vi "Auto Angle.vi"(9 "Yaw":T10 scale format="%.3f", 10 "Rotation PID Config":T2 {"Max I Accu"."Low" format="%#.8f"; "Max I Accu"."High" format="%#.8f"; "Gains"."F" format="%#.8f"; "Gains"."D" format="%#.8f"; "Gains"."I" format="%#.8f"; "Gains"."P" format="%#.8f"; "Error Allowed"."Low" format="%#.8f"; "Error Allowed"."High" format="%#.8f"; "I Zone"."Low" format="%#.8f"; "I Zone"."High" format="%#.8f"; "Max Out"."REV" format="%.2f"; "Max Out"."FWD" format="%.2f"}, 11 "CMD_ACT_SwerveDrive_Data in":T6 {"Auto Angle" scale format="%.3f"; "Direction"."Rotate(Yaw) CCW 1 CW -1" scale=1.0..-1.0; "Direction"."Traverse"."Angle" scale format="%.3f"; "Direction"."Traverse"."Velocity" scale=-1.0..1.0 scale format="%.1f"}) -> (1 "At Angle":bool, 3 "CMD_ACT_SwerveDrive_Data out":T6 {"Auto Angle" scale format="%.3f"; "Direction"."Rotate(Yaw) CCW 1 CW -1" scale=1.0..-1.0; "Direction"."Traverse"."Angle" scale format="%.3f"; "Direction"."Traverse"."Velocity" scale=-1.0..1.0 scale format="%.1f"})   [LabVIEW 2023, in "Thor-SwerveDrive_ACT.lvlib"]
uses:
  Thor-SwerveDrive_ACT.lvlib
  Shared Code/TypeDefs/Dial_Compase heading unit circle CCW positive.ctl
  Shared Code/TypeDefs/ENUM_Swerve_CMD_Mode Select.ctl
  Shared Code/TypeDefs/Level_Velocity plus-minus 1.ctl
  Shared Code/TypeDefs/Cluster_Module Velocity-Direction-Rotations.ctl
  Type Defs/NUM_Rotate Input.ctl
  Shared Code/TypeDefs/Cluster_CMD_Direction Data.ctl
  Shared Code/TypeDefs/Cluster_X-Y.ctl
  Cluster_CMD_ACT_Data.ctl
  Shared Code/TypeDefs/Cluster_FWD  REV Values.ctl
  Shared Code/TypeDefs/Cluster_High-Low.ctl
  Shared Code/TypeDefs/Cluster_PID Gains.ctl
  Shared Code/TypeDefs/Cluster_PID Config.ctl
panel:
  out "Mode":T1
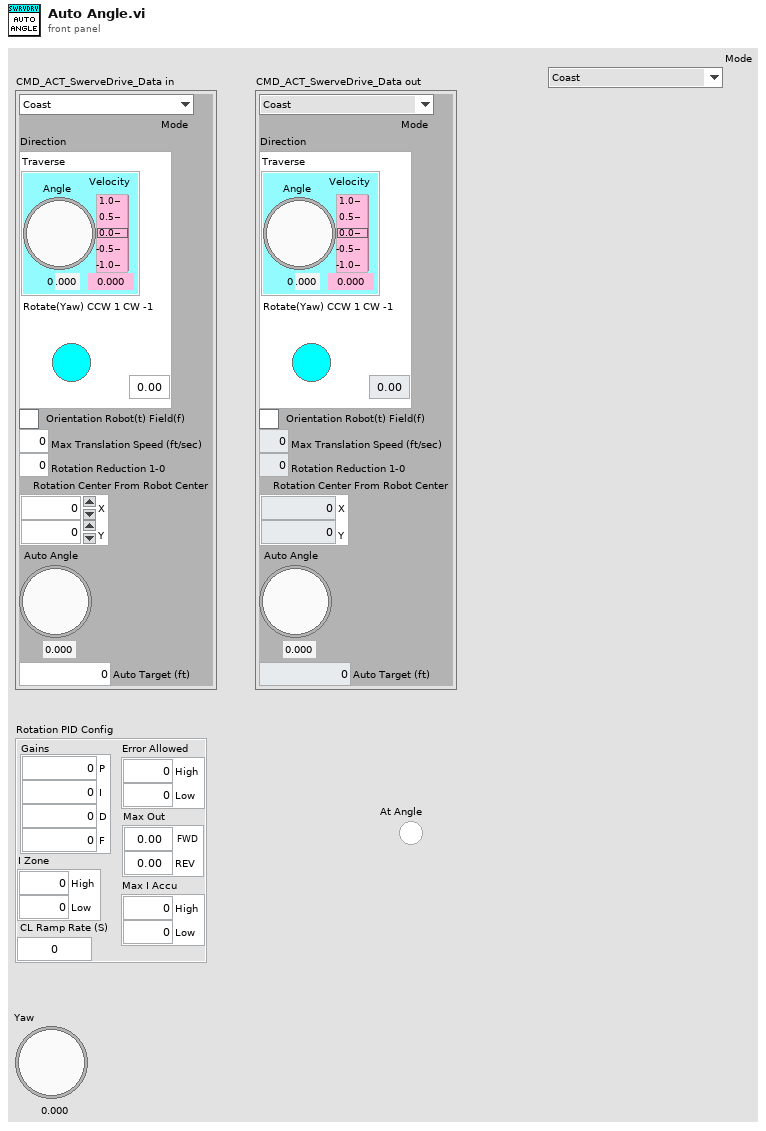
[diagram p1: front panel]
types:
  T1 = typedef "ENUM_Swerve_CMD_Mode Select.ctl" = enum16{"Coast", "Manual", "Auto Trans Auto Rotate", "Manual Trans Auto Rotate", "Balance", "Stop Brake", "Lock Wheels"}
  T2 = typedef "Cluster_PID Config.ctl" = cluster{"Gains":T3, "Error Allowed":T4, "I Zone":T4, "Max Out":T5, "Max I Accu":T4, "CL Ramp Rate (S)":dbl}
  T3 = typedef "Cluster_PID Gains.ctl" = cluster{"P":dbl, "I":dbl, "D":dbl, "F":dbl}
  T4 = typedef "Cluster_High-Low.ctl" = cluster{"High":dbl, "Low":dbl}
  T5 = typedef "Cluster_FWD  REV Values.ctl" = cluster{"FWD":dbl, "REV":dbl}
  T6 = typedef "Thor-SwerveDrive_ACT.lvlib/Cluster_CMD_ACT_Data.ctl" = cluster{"Mode":T1, "Direction":T7, "Orientation Robot(t) Field(f)":bool, "Max Translation Speed (ft/sec)":dbl, "Rotation Reduction 1-0":dbl, "Rotation Center From Robot Center":T12, "Auto Angle":T10, "Auto Target (ft)":dbl}
  T7 = typedef "Cluster_CMD_Direction Data.ctl" = cluster{"Traverse":T8, "Rotate(Yaw) CCW 1 CW -1":T11}
  T8 = typedef "Cluster_Module Velocity-Direction-Rotations.ctl" = cluster{"Velocity":T9, "Angle":T10, "Rotations Count":dbl}
  T9 = typedef "Level_Velocity plus-minus 1.ctl" = dbl
  T10 = typedef "Dial_Compase heading unit circle CCW positive.ctl" = dbl
  T11 = typedef "NUM_Rotate Input.ctl" = dbl
  T12 = typedef "Cluster_X-Y.ctl" = cluster{"X":dbl, "Y":dbl}
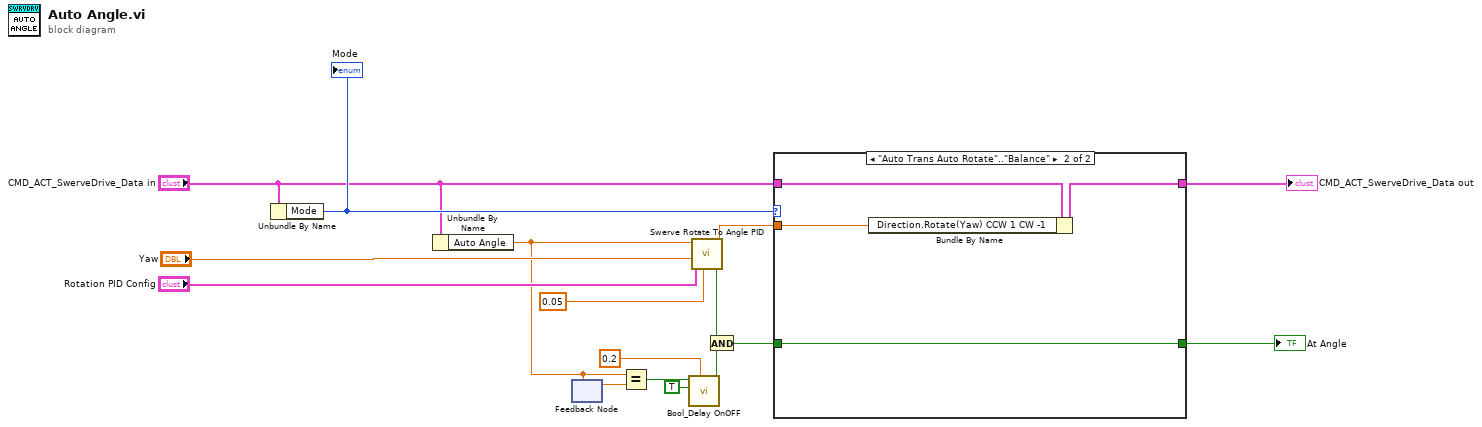
[diagram p0: block diagram]
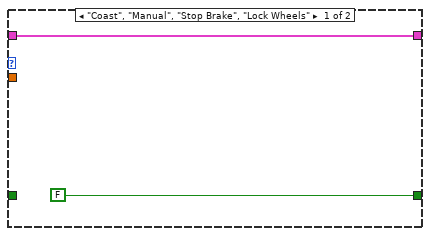
[diagram p2: hidden frame]
diagram:
  n1 = Unbundle By Name("CMD_ACT_SwerveDrive_Data in") -> ("Mode"=w14:T1)
  "Mode" <- w14
  n2 = Unbundle By Name("CMD_ACT_SwerveDrive_Data in") -> ("Auto Angle"=w8:T10)
  n3 = feedback #1() -> (w9:T10)  [unwired: 1 in]
  n4 = feedback-in #1(w8) -> ()
  n5 = Equal?(x=w8, y=w9) -> (x = y?=w7:bool)
  n6 = call "Bool_Delay OnOFF.vi"("Delay Time(S)"=0.2, "Delay On(t) Off(f)"=TRUE, "Input"=w7) -> ("Output"=w4:bool)  [unwired: 7 in, 1 out]
  n7 = call "Swerve Rotate To Angle PID.vi"("Target Cycle Time(S)"=0.05, "PID Config"="Rotation PID Config", "Current Yaw"="Yaw", "Target Yaw"=w8) -> ("At Angle Out"=w3:bool, "Direction.Rotate(Yaw) CCW 1 CW -1 Out"=w10:T11)  [unwired: 5 in, 1 out]
  n8 = And(x=w3, y=w4) -> (x .and. y?=w2:bool)
  n9 = case shown="\"Auto Trans Auto Rotate\"..\"Balance\"" w14 {
    tunnel: "CMD_ACT_SwerveDrive_Data in" -> [w18 w22]
    tunnel: w10 -> [_ w21]
    tunnel: [w18 w20] -> w12
    tunnel: w2 -> [_ w19]
    tunnel: [FALSE w19] -> w1
    frame "Coast", "Manual", "Stop Brake", "Lock Wheels" {
    }
    frame "Auto Trans Auto Rotate".."Balance" {
      n10 = Bundle By Name(cluster=w22, "Direction.Rotate(Yaw) CCW 1 CW -1"=w21) -> (w20:T6)
    }
  }
  "CMD_ACT_SwerveDrive_Data out" <- w12
  "At Angle" <- w1
